vi "Read Message.vi"(6 "timeout in ms (100)":i32=100, 8 "error in (no error)":errorcluster, 10 "index":i32, 11 "RemoteControl in":refnum<class "RemoteControl.lvclass">) -> (0 "error out":errorcluster, 1 "Data":variant, 2 "Command":string, 3 "RemoteControl out":refnum<class "RemoteControl.lvclass">, 4 "ID":string)   [LabVIEW 2019, in "RemoteControl.lvclass"]
uses:
  RemoteControl.lvclass
  Typedefs/Message--Cluster.ctl
  Private/RemoteControlGlobal.vi
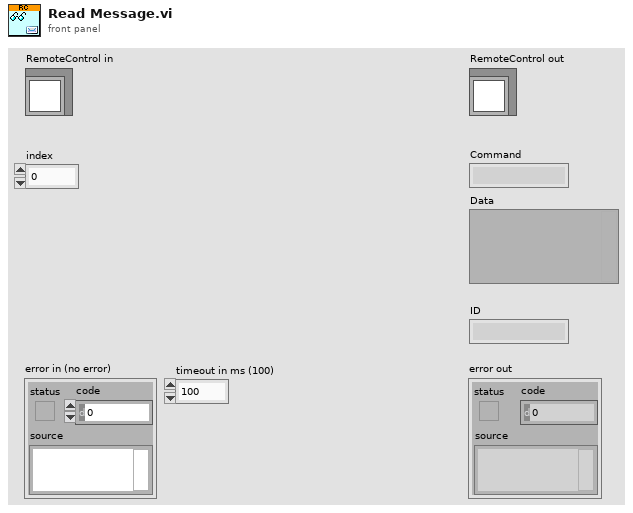
[diagram p1: front panel]
types:
  T1 = typedef "RemoteControl.lvclass/Message--Cluster.ctl" = cluster{"Command":string, "Data":variant, "ID":string}
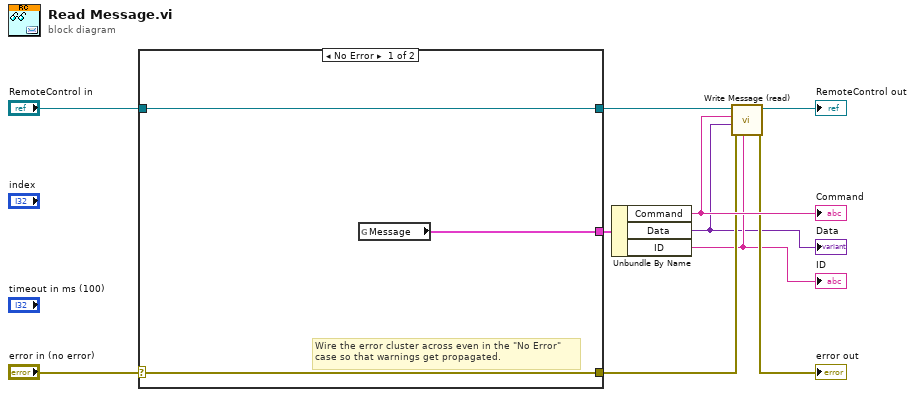
[diagram p0: block diagram]
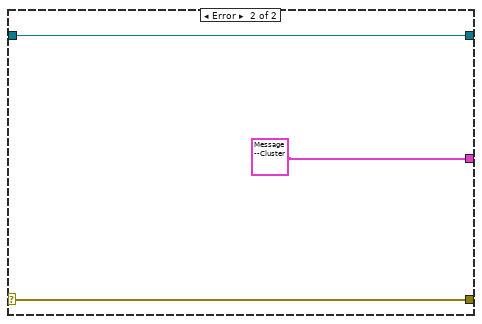
[diagram p2: hidden frame]
diagram:
  n1 = case shown="No Error" "error in (no error)" {
    selector: "error in (no error)" -> [w13 w16]
    tunnel: [w13 w16] -> w4
    tunnel: [w11 w15] -> w6
    tunnel: "RemoteControl in" -> [w11 w15]
    tunnel: [w12 T1 {"Command"="", "Data"=variant, "ID"=""} ("Message")] -> w8
    frame No Error {
      # "Wire the error cluster across even in the \"No Error\"\ncase so that warnings get propagated."
      n2 = global read "RemoteControlGlobal.vi" "Message"() -> (w12:T1)
    }
    frame Error {
    }
  }
  n3 = Unbundle By Name(w8) -> ("Command"=w5:string, "Data"=w1:variant, "ID"=w2:string)
  "ID" <- w2
  "Command" <- w5
  "Data" <- w1
  n4 = call "Write Message (read).vi"("ID (Read)"=w2, "error in (no error)"=w4, "Data (Read)"=w1, "Command (Read)"=w5, "RemoteControl in"=w6) -> ("error out"=→"error out":errorcluster, "RemoteControl out"=→"RemoteControl out":refnum<class "RemoteControl.lvclass">)  [unwired: 5 in]
